vi "add.vi"(8 "error in (no error)":errorcluster, 10 "Composite Employee.lvclass":refnum<class "Composite Employee.lvclass">, 11 "Composite Employee in":refnum<class "Composite Employee.lvclass">) -> (0 "error out":errorcluster, 3 "Composite Employee out":refnum<class "Composite Employee.lvclass">)   [LabVIEW 2018, in "Composite Employee.lvclass"]
uses:
  Composite Employee.lvclass
  C:/Users/fflores/Documents/LabVIEW-Open-Projects/LabIVEW OOP Design Patterns/Composite Pattern/Employee Class/Employee.lvclass
  Composite Employee.lvclass/Composite Employee.ctl
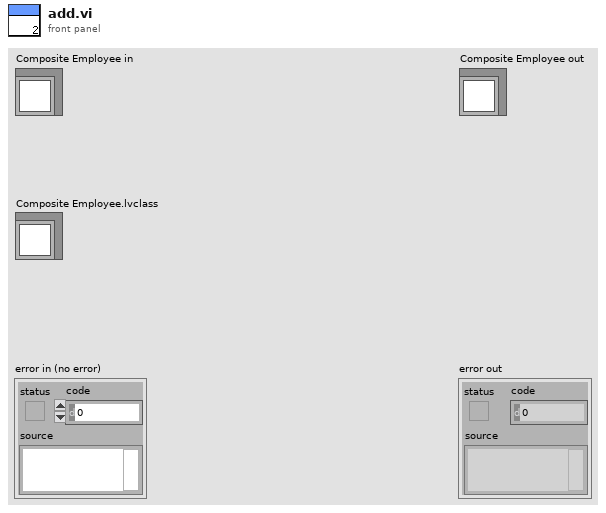
[diagram p1: front panel]
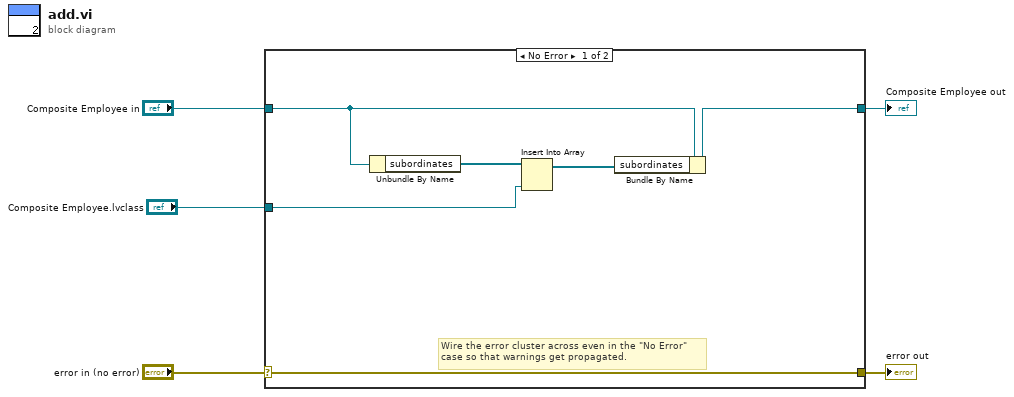
[diagram p0: block diagram]
diagram:
  n1 = case shown="No Error" "error in (no error)" {
    selector: "error in (no error)" -> [w11 w13]
    tunnel: [w11 w13] -> w4
    tunnel: [w10 w12] -> w2
    tunnel: "Composite Employee in" -> [w9 w12]
    tunnel: "Composite Employee.lvclass" -> [w6 _]
    frame No Error {
      # "Wire the error cluster across even in the \"No Error\"\ncase so that warnings get propagated."
      n2 = Unbundle By Name(w9) -> ("subordinates"=w8:refnum<class "Employee.lvclass">[])
      n3 = Insert Into Array(array=w8, new element=w6) -> (w7:refnum<class "Employee.lvclass">[])  [unwired: 1 in]
      n4 = Bundle By Name(cluster=w9, "subordinates"=w7) -> (w10:refnum<class "Composite Employee.lvclass">)
    }
    frame Error {
    }
  }
  "error out" <- w4
  "Composite Employee out" <- w2
